vi "Set IO Direction.vi"(10 "iDirection":i32, 11 "index":i32) -> (3 "function return":u32)   [LabVIEW 2018, in "Copy of Andor SDK.lvlib"]
doc: "EXPNETTYPE unsigned int WINAPI SetIODirection(int index, int iDirection);"
uses:
  Copy of Andor SDK.lvlib
  <userlib>/Andor SDK/ATMCD32D.dll
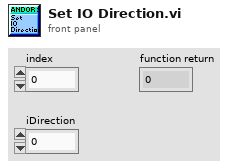
[diagram p1: front panel]
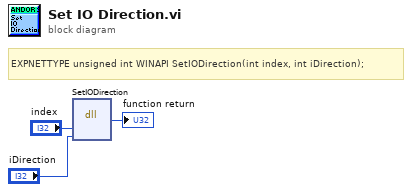
[diagram p0: block diagram]
diagram:
  # "EXPNETTYPE unsigned int WINAPI SetIODirection(int index, int iDirection);"
  n1 = dll-call lib="C:/Program Files (x86)/National Instruments/LabVIEW 2018/user.lib/Andor SDK/ATMCD32D.*" fn="SetIODirection"("index"="index", "iDirection"="iDirection") -> (→"function return":u32)  [unwired: 5 in, 2 out]
